vi "extract queue to time range 1 element.vi"(6 "most recent?":bool, 7 "recent interval":dbl=5.0, 8 "error in (no error)":errorcluster, 9 "t0":dbl=-1.0, 10 "t1":dbl=-1.0, 11 "queue":T1) -> (0 "error out":errorcluster, 2 "extracted data":T2[](array[typedef]))   [LabVIEW 2017]
uses:
  typedefs/reading1.ctl
  typedefs/reading 1 queue.ctl
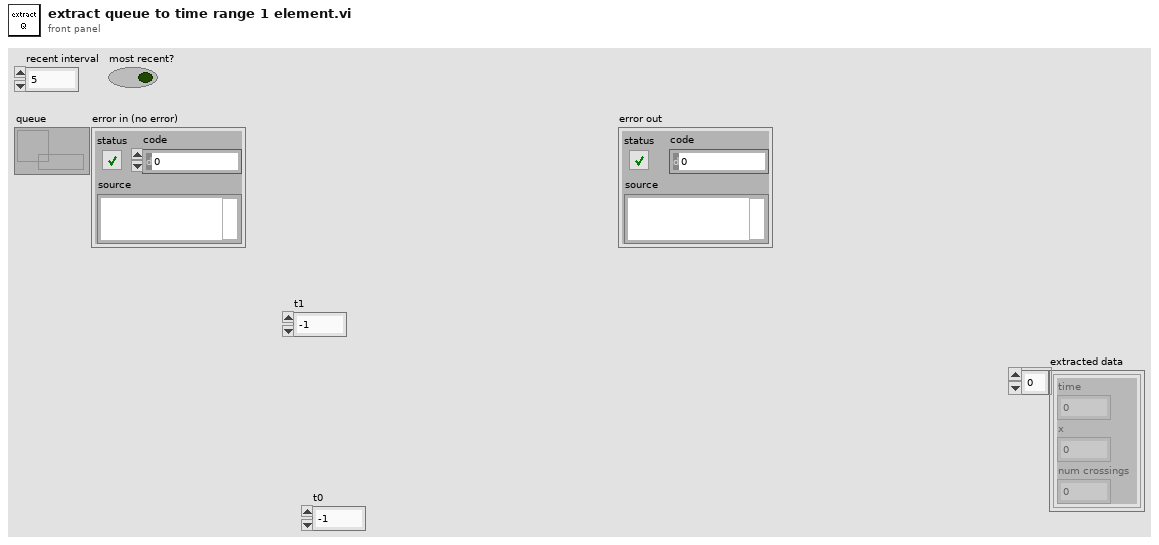
[diagram p1: front panel]
types:
  T1 = typedef "reading 1 queue.ctl" = refnum<queue>
  T2 = typedef "reading1.ctl" = cluster{"time":dbl, "x":dbl, "num crossings":u32}
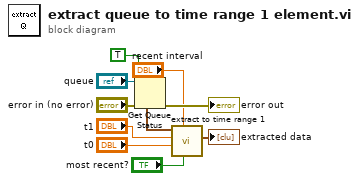
[diagram p0: block diagram]
diagram:
  n1 = Get Queue Status(queue="queue", return elements? (F)=TRUE, error in (no error)="error in (no error)") -> (error out=→"error out":errorcluster, elements=w7:T2[])  [unwired: 6 out]
  n2 = call "extract to time range 1.vi"("most recent?"="most recent?", "recent interval"="recent interval", "t0"="t0", "t1"="t1", "elements"=w7) -> ("extracted data"=→"extracted data":T2[])  [unwired: 6 in]
